vi "User Access Level FGV.vi"(7 "User Level Control":T1, 8 "Error In":errorcluster, 10 "User Name":string) -> (0 "Error Out":errorcluster, 1 "User Level":string)   [LabVIEW 2024]
doc: "This FGV holds the Access Level for the user currently logged in. It executes the following methods:\n\n1. <B>Read User Access Level File:</B> Reads a tab-delimited text file containing User Names and corresponding Access Levels.\n2. <B>Set Current Access Level:</B> Sets the Access level for the User Name input.\n3. <B>Get Current Access Level:</B> Returns the Access level for the current User."
uses:
  User Level Cmd.ctl
  <vilib>/Utility/file.llb/Read Delimited Spreadsheet (string).vi
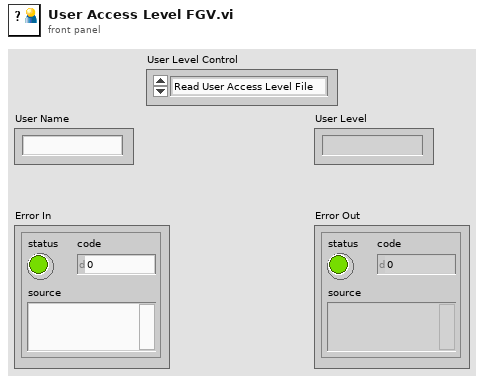
[diagram p1: front panel]
types:
  T1 = typedef "User Level Cmd.ctl" = enum16{"Read User Access Level File", "Set Current Access Level", "Get Current Access Level"}
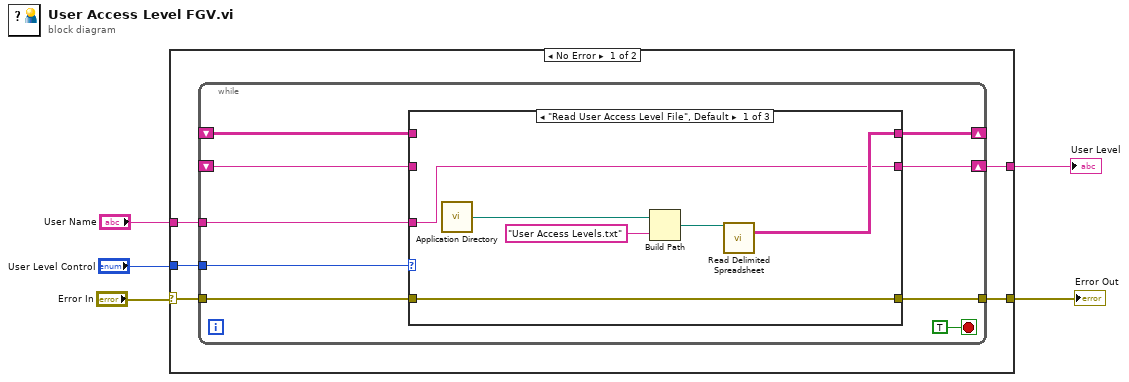
[diagram p0: block diagram]
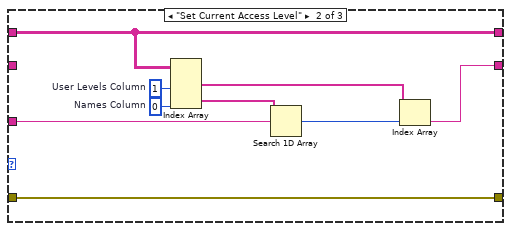
[diagram p2: hidden frame]
diagram:
  n1 = case shown="No Error" "Error In" {
    selector: "Error In" -> [w9 w39]
    tunnel: "User Level Control" -> [w10 _]
    tunnel: [w8 w39] -> w3
    tunnel: [w7 w38] -> w1
    tunnel: "User Name" -> [w6 w38]
    frame No Error {
      n2 = while {
        tunnel: w10 -> [w18]
        tunnel: w9 -> [w17]
        tunnel: [w16] -> w8
        shift-right: [w15] -> _
        shift-left: _ -> [w14]
        shift-right: [w12] -> w7
        shift-left: _ -> [w13]
        tunnel: w6 -> [w11]
        stop <- TRUE stop-if-true
        n3 = case shown="\"Read User Access Level File\", Default" w18 {
          tunnel: [w20 w34 w35] -> w16
          tunnel: w17 -> [w20 w34 w35]
          tunnel: [w22 w31 w37] -> w15
          tunnel: w14 -> [_ w31 w37]
          tunnel: w13 -> [_ _ w36]
          tunnel: [w21 w33 w36] -> w12
          tunnel: w11 -> [w21 w27 _]
          frame "Read User Access Level File", Default {
            n4 = call <vilib>:"Application Directory.vi"() -> ("Application Directory"=w24:path)
            n5 = Build Path(base path=w24, name or relative path="User Access Levels.txt") -> (appended path=w23:path)
            n6 = call-poly <vilib>:"Read Delimited Spreadsheet.vi"("file path (dialog if empty)"=w23) -> ("all rows"=w22:string[][])  [unwired: 9 in, 5 out]
          }
          frame "Set Current Access Level" {
            w29 = 0  # Names Column
            w30 = 1  # User Levels Column
            n7 = Index Array "Index Array"(array=w31, index (col) #1=w30, index (col) #2=w29) -> (element #1=w26:string[], element #2=w28:string[])  [unwired: 2 in]
            n8 = Search 1D Array(1D array=w28, element=w27) -> (index of element=w32:i32)  [unwired: 1 in]
            n9 = Index Array "Index Array"(array=w26, index=w32) -> (element=w33:string)
          }
          frame "Get Current Access Level" {
          }
        }
      }
    }
    frame Error {
    }
  }
  "User Level" <- w1
  "Error Out" <- w3
